vi "array -- bilinear regression.vi"(7 "action":T1=enum."calc", 9 "fit":dbl[](array[numeric]), 10 "y":dbl[](array[numeric]), 11 "x":dbl[](array[numeric])) -> (1 "fit OUT":dbl[](array[numeric]), 2 "y OUT":dbl[](array[numeric]), 3 "x OUT":dbl[](array[numeric]))   [LabVIEW 2020]
uses:
  array -- fit control .ctl
  <vilib>/Analysis/baseanly.llb/Real A x B.vi
  <vilib>/Analysis/baseanly.llb/Real Inverse Matrix.vi
  <vilib>/Analysis/Matrix/Numeric/Conversions/Matrix To Array - RM.vi
  <vilib>/Analysis/NI_AALBase.lvlib
  <vilib>/Analysis/Matrix/NI_Matrix.lvlib
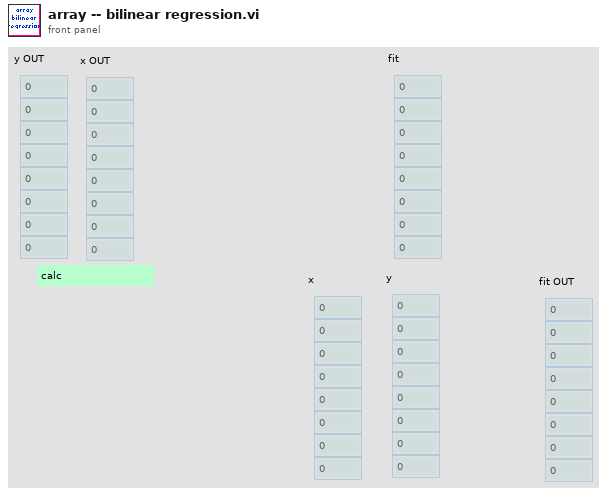
[diagram p1: front panel]
types:
  T1 = typedef "array -- fit control .ctl" = enum16{"fit", "calc", "check", "init"}
  T2 = typedef "NI_Matrix.lvlib/RealMatrix.ctl" = dbl[][]
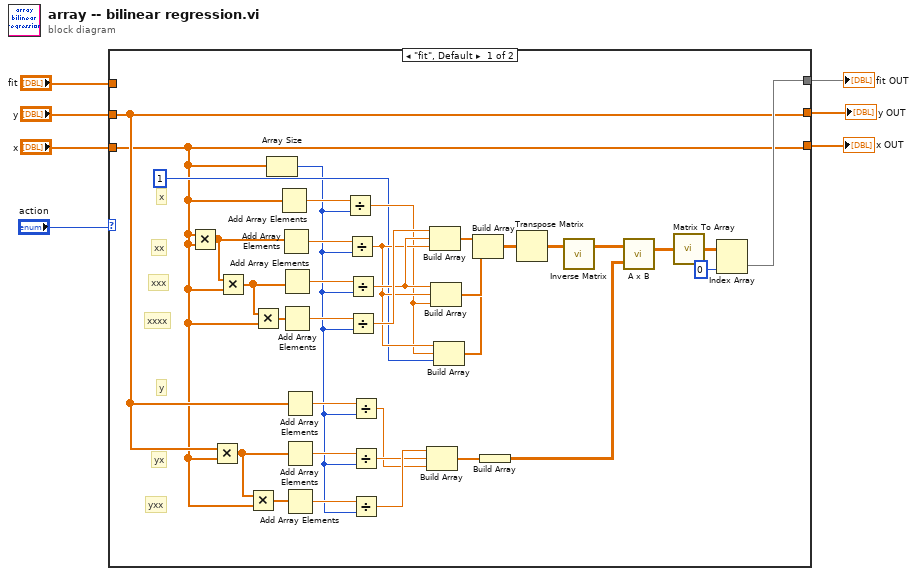
[diagram p0: block diagram]
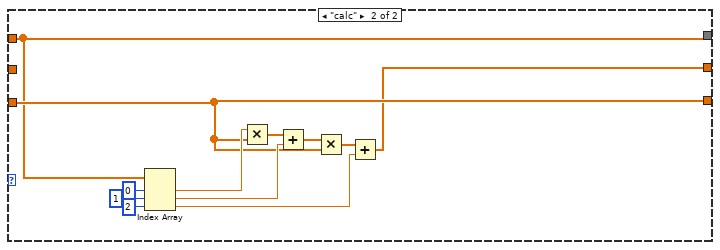
[diagram p2: hidden frame]
diagram:
  n1 = case shown="\"fit\", Default" "action" {
    tunnel: "y" -> [w9 _]
    tunnel: "x" -> [w8 w45]
    tunnel: [w14 w43] -> w5
    tunnel: [w9 w44] -> w4
    tunnel: [w8 w45] -> w3
    tunnel: "fit" -> [_ w43]
    frame "fit", Default {
      # "yxx"
      # "yx"
      # "y"
      # "xxxx"
      # "xxx"
      # "xx"
      # "x"
      n2 = Multiply(x=w8, y=w8) -> (x*y=w13:dbl[])
      n3 = Multiply(x=w9, y=w8) -> (x*y=w24:dbl[])
      n4 = Multiply(x=w13, y=w8) -> (x*y=w38:dbl[])
      n5 = Multiply(x=w24, y=w8) -> (x*y=w23:dbl[])
      n6 = Multiply(x=w38, y=w8) -> (x*y=w37:dbl[])
      n7 = Array Size(array=w8) -> (size(s)=w25:i32)
      n8 = Add Array Elements(numeric array=w8) -> (sum=w41:dbl)
      n9 = Add Array Elements(numeric array=w13) -> (sum=w42:dbl)
      n10 = Add Array Elements(numeric array=w38) -> (sum=w40:dbl)
      n11 = Add Array Elements(numeric array=w37) -> (sum=w39:dbl)
      n12 = Add Array Elements(numeric array=w9) -> (sum=w28:dbl)
      n13 = Add Array Elements(numeric array=w24) -> (sum=w27:dbl)
      n14 = Add Array Elements(numeric array=w23) -> (sum=w26:dbl)
      n15 = Divide(x=w41, y=w25) -> (x/y=w33:dbl)
      n16 = Divide(x=w42, y=w25) -> (x/y=w34:dbl)
      n17 = Divide(x=w40, y=w25) -> (x/y=w35:dbl)
      n18 = Divide(x=w39, y=w25) -> (x/y=w36:dbl)
      n19 = Divide(x=w28, y=w25) -> (x/y=w20:dbl)
      n20 = Divide(x=w27, y=w25) -> (x/y=w21:dbl)
      n21 = Divide(x=w26, y=w25) -> (x/y=w22:dbl)
      n22 = Build Array(w22, w21, w20) -> (w19:dbl[])
      n23 = Build Array(w36, w35, w34) -> (w31:dbl[])
      n24 = Build Array(w35, w34, w33) -> (w30:dbl[])
      n25 = Build Array(w34, w33, 1) -> (w29:dbl[])
      n26 = Build Array(w31, w30, w29) -> (w11:T2)
      n27 = Build Array(w19) -> (w12:T2)
      n28 = Transpose Matrix(1:w11) -> (0:w10:T2)
      n29 = call-poly <vilib>:"Inverse Matrix.vi"("Input Matrix"=w10) -> ("Inverse Matrix"=w18:T2)  [unwired: 1 in, 1 out]
      n30 = call-poly <vilib>:"A x B.vi"("B"=w12, "A"=w18) -> ("A x B"=w17:T2)  [unwired: 1 out]
      n31 = call-poly <vilib>:"Matrix To Array.vi"("Real Matrix"=w17) -> ("Real 2D Array"=w16:dbl[][])
      n32 = Index Array(array=w16, index (col)=0 ("disabled index (col)")) -> (element=w14:dbl[])  [unwired: 1 in]
    }
    frame "calc" {
      n33 = Index Array(array=w43, index #1=0 ("index"), index #2=1 ("index"), index #3=2 ("index")) -> (element #1=w51:dbl, element #2=w49:dbl, element #3=w46:dbl)
      n34 = Multiply(x=w51, y=w45) -> (x*y=w50:dbl[])
      n35 = Add(x=w50, y=w49) -> (x+y=w48:dbl[])
      n36 = Multiply(x=w48, y=w45) -> (x*y=w47:dbl[])
      n37 = Add(x=w47, y=w46) -> (x+y=w44:dbl[])
    }
  }
  "fit OUT" <- w5
  "y OUT" <- w4
  "x OUT" <- w3
